vi "Get Handle And Command.vi"(7 "Error In":errorcluster, 10 "Command":string="status") -> (0 "Error Out":errorcluster, 2 "Command URL":string, 3 "RedEdge client handle out":T1)   [LabVIEW 2014]
uses:
  <vilib>/httpClient/ClientHandle.ctl
  <vilib>/httpClient/LabVIEWHTTPClient.lvlib
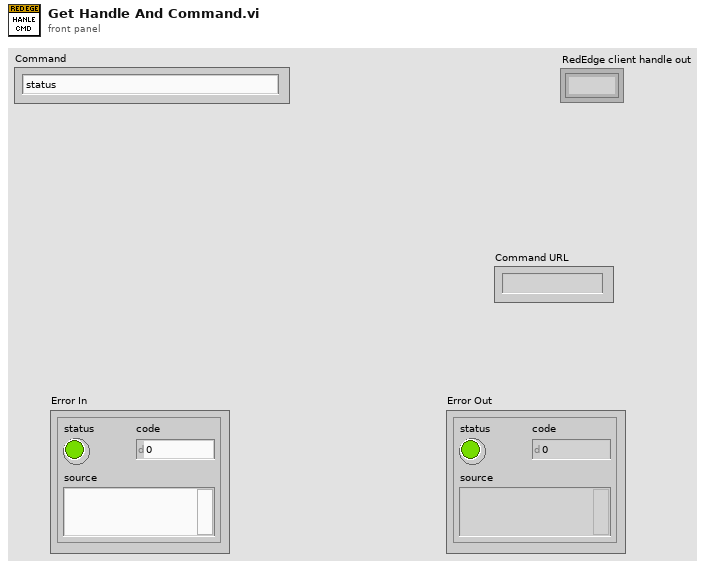
[diagram p1: front panel]
types:
  T1 = typedef "LabVIEWHTTPClient.lvlib/ClientHandle.ctl" = refnum<k1>
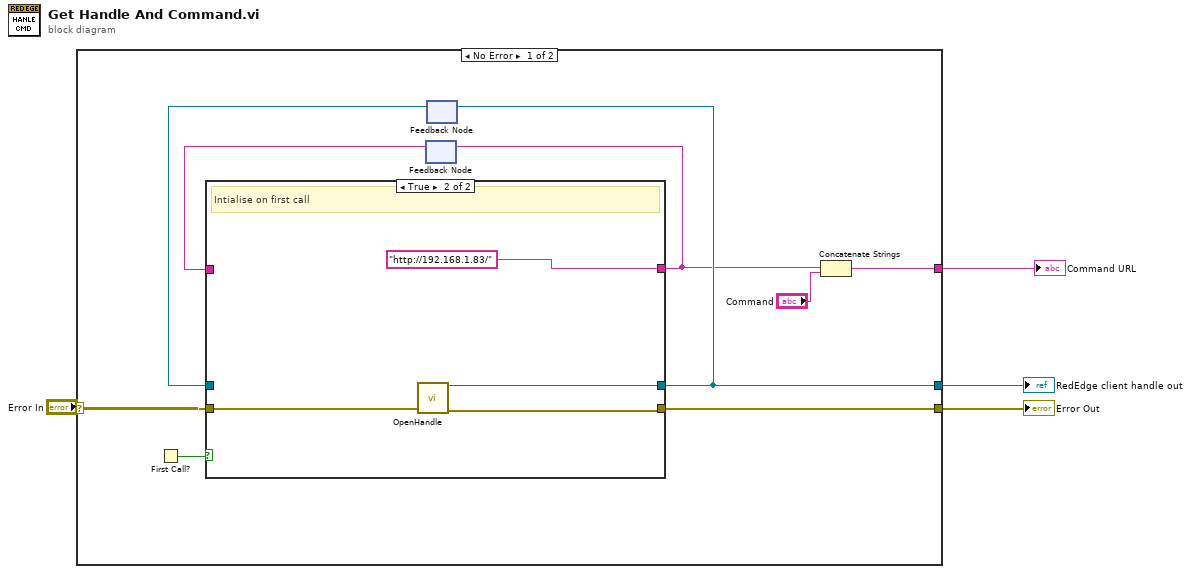
[diagram p0: block diagram]
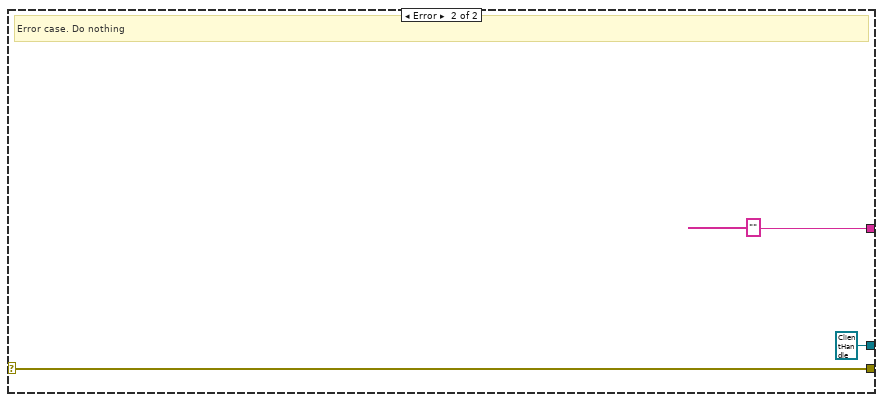
[diagram p3: hidden frame]
diagram:
  n1 = case shown="No Error" "Error In" {
    selector: "Error In" -> [w13 w21]
    tunnel: [w5 w21] -> w3
    tunnel: [w7 "" ("url")] -> w2
    tunnel: [w11 T1 refnum ("client handle out")] -> w1
    frame No Error {
      n2 = First Call?() -> (First Call?: T/F=w12:bool)
      n3 = feedback #1() -> (w10:string)  [unwired: 1 in]
      n4 = feedback #2() -> (w9:T1)  [unwired: 1 in]
      n5 = case shown="True" w12 {
        tunnel: [w14 "http://192.168.1.83/" ("url")] -> w6
        tunnel: w13 -> [w15 w18]
        tunnel: [w15 w17] -> w5
        tunnel: [w16 w19] -> w11
        tunnel: w10 -> [w14 _]
        tunnel: w9 -> [w16 _]
        frame False {
        }
        frame True {
          # "Intialise on first call"
          n6 = call <vilib>:"OpenHandle.vi"("error in (no error)"=w18) -> ("client handle out"=w19:T1, "error out"=w17:errorcluster)  [unwired: 13 in]
        }
      }
      n7 = feedback-in #1(w6) -> ()
      n8 = feedback-in #2(w11) -> ()
      n9 = Concatenate Strings(w6, "Command") -> (w7:string)
    }
    frame Error {
      # "Error case. Do nothing"
    }
  }
  "Error Out" <- w3
  "Command URL" <- w2
  "RedEdge client handle out" <- w1
